vi "Pre Launch Init.vi"(11 "IViewModel In":refnum<class "IViewModel.lvclass">) -> (0 "error out":errorcluster, 3 "IViewModel Out":refnum<class "IViewModel.lvclass">)   [LabVIEW 2020, in "IViewModel.lvlib" / "IViewModel.lvclass"]
doc: "(<B>Filename</B>: Actor Framework.lvlib:Actor.lvclass:Pre Launch Init.vi)\n\nDefines behavior that occurs after the Launch Nested Actor method is invoked but before the actor's Actor Core method begins running.\n\nBy default, this method does nothing. A descendant class may override it to define behavior.\n\n<License>\nCopyright © 2017 Composed Systems, LLC | All rights reserved\nwww.composed.io\n\nAuthor: Ethan Stern <ethan.stern@composed.io>\n\nThis software is provided \"AS IS\" WITHOUT WARRANTIES, either express or implied, AND IS FOR EDUCATIONAL PURPOSES ONLY.\n</License>"
uses:
  IViewModel.lvclass
  C:/Program Files/National Instruments/LabVIEW 2020/vi.lib/ActorFramework/Actor/Actor.lvclass
  <vilib>/ActorFramework/Actor/Actor.lvclass/Actor.ctl
  <vilib>/ActorFramework/Message Enqueuer/Message Enqueuer.lvclass/Message Enqueuer.ctl
  <vilib>/ActorFramework/Message Enqueuer/Message Priority.ctl
  composed-event-logger/Source/Composed Log/Types/Log Level.ctl
  mva-core/Source/IObserver/IObserver/IObserver.lvclass/IObserver.ctl
  composed-event-logger/Source/Composed Log/LoggerReference/LoggerReference.lvclass/LoggerReference.ctl
  IViewModel.lvclass/IViewModel.ctl
  IViewable/IViewable/IViewable.lvclass/IViewable.ctl
  <vilib>/ActorFramework/Message Enqueuer/Init from Existing Queue.vi
  <vilib>/ActorFramework/Message Enqueuer/Enqueue.vi
  composed-event-logger/Source/Composed Log/LoggerReference/Log Event.vi
  composed-event-logger/Source/Composed Log/LoggerReference/Log.vi
  composed-event-logger/Source/Composed Log/LoggerReference/Get Valid Event Time.vi
  composed-event-logger/Source/Composed Log/LoggerReference/Remove Stale Logs.vi
  IViewModel Messages/Launch Root Model Msg/Launch Root Model Msg.lvclass
  C:/Program Files/National Instruments/LabVIEW 2020/vi.lib/ActorFramework/Message/Message.lvclass
  <vilib>/ActorFramework/Message Priority Queue/Priority Enqueue.vi
  <vilib>/Utility/LVClass/Get LV Class Name.vi
  <vilib>/ActorFramework/Message Enqueuer/Message Enqueuer.lvclass
  IViewManager/IViewManager/IViewManager.lvclass
  <vilib>/ActorFramework/Actor/Actor.lvclass
  IViewable/IViewable/IViewable.lvclass
  IViewable/ApplicationStyleReference/ApplicationStyleReference.lvclass
  mva-core/Source/IObserver/IObserver/IObserver.lvclass
  composed-event-logger/Source/Composed Log/Composed Log.lvlib
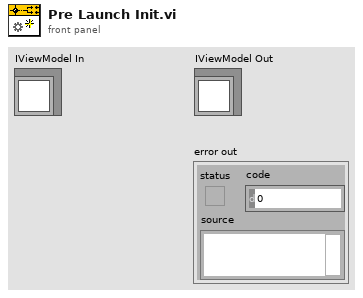
[diagram p1: front panel]
types:
  T1 = typedef "Actor Framework.lvlib/Message Enqueuer.lvclass/Message Priority.ctl" = enum16{"Low", "Normal", "High"}
  T2 = typedef "Composed Log.lvlib/Log Level.ctl" = enum16{"Debug", "Info", "Warning", "Error", "Critical"}
  T3 = typedef "IViewable.lvlib/ApplicationStyleReference.lvclass/Application Style Reference.ctl" = refnum<data-value>
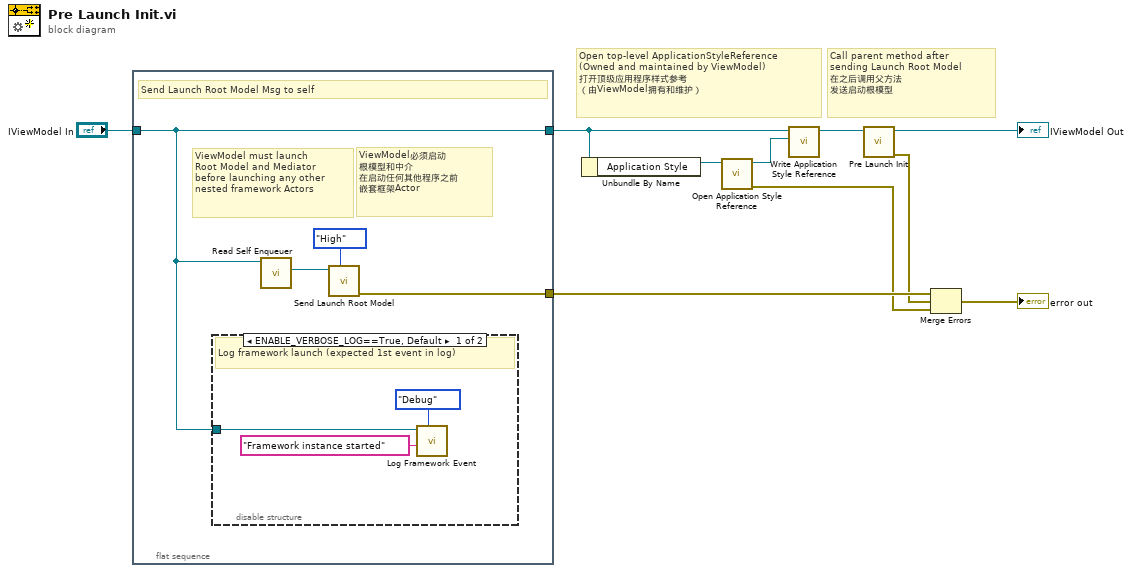
[diagram p0: block diagram]
diagram:
  # "Call parent method after\nsending Launch Root Model\n在之后调用父方法\n发送启动根模型"
  # "Open top-level ApplicationStyleReference\n(Owned and maintained by ViewModel)\n打开顶级应用程序样式参考\n（由ViewModel拥有和维护）"
  n1 = flat-sequence {
    tunnel: [w13] -> w10
    tunnel: "IViewModel In" -> [w11]
    tunnel: [w11] -> w2
    frame #0 {
      # "ViewModel必须启动\n根模型和中介\n在启动任何其他程序之前\n嵌套框架Actor"
      # "ViewModel must launch\nRoot Model and Mediator\nbefore launching any other\nnested framework Actors"
      # "Send Launch Root Model Msg to self"
      n2 = disable-structure shown="ENABLE_VERBOSE_LOG==True, Default" {
        disable-tunnel: w11 -> [w16 _]
        frame condition #0 (active) {
          # "Log framework launch (expected 1st event in log)"
          n3 = call "Log Framework Event.vi"("Event Level (Debug)"=Log_Level."Debug", "Data To Log"="Framework instance started", "IObserver in"=w16) -> ()  [unwired: 8 in, 1 out]
        }
        frame condition #1 {
          # "Remove all logging from this method at compile time"
        }
      }
      n4 = call <vilib>:"Read Self Enqueuer.vi"("Actor"=w11) -> ("Self Enqueuer"=w14:refnum<class "Message Enqueuer.lvclass">)  [unwired: 10 in]
      n5 = call "Send Launch Root Model.vi"("Message Priority (Normal)"=Message_Priority."High", "Message Enqueuer"=w14) -> ("error out"=w13:errorcluster)  [unwired: 8 in, 1 out]
    }
  }
  n6 = Unbundle By Name(w2) -> ("Application Style"=w8:refnum<class "IApplicationStyle.lvclass">)
  n7 = call "Open Application Style Reference.vi"("ApplicationStyle"=w8) -> ("error out"=w5:errorcluster, "Application Style Reference"=w7:T3)  [unwired: 9 in]
  n8 = call "Write Application Style Reference.vi"("Application Style Reference"=w7, "IViewable in"=w2) -> ("IViewable out"=w9:refnum<class "IViewModel.lvclass">)  [unwired: 9 in]
  n9 = call-parent "Pre Launch Init.vi"("IViewManager in"=w9) -> ("error out"=w1:errorcluster, "IViewManager out"=→"IViewModel Out":refnum<class "IViewModel.lvclass">)  [unwired: 9 in]
  n10 = Merge Errors(w10, w1, w5) -> (→"error out":errorcluster)
